vi "Configuration Reference.vi"(8 "Error in":errorcluster, 11 "INL DNL Test in":refnum<class "INL DNL Test.lvclass">) -> (0 "Error out":errorcluster, 2 "VI Ref":refnum<vi>, 3 "INL DNL Test out":refnum<class "INL DNL Test.lvclass">)   [LabVIEW 2020, in "INL DNL Test.lvclass"]
doc: "Runs the configuration page asynchronously."
uses:
  INL DNL Test.lvclass
  Parent/Typedef/LV2 Control.ctl
  Configuration Page.vi
  Parent/Test.lvclass
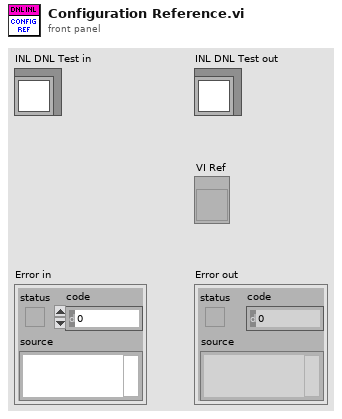
[diagram p1: front panel]
types:
  T1 = typedef "Test.lvclass/LV2 Control.ctl" = enum16{"Home", "Mode", "Config", "Status", "Read"}
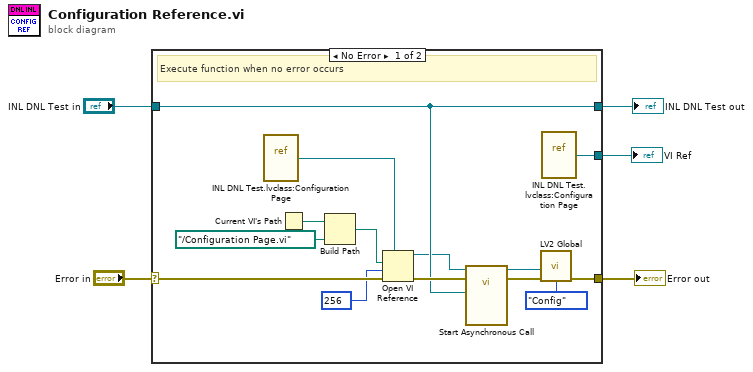
[diagram p0: block diagram]
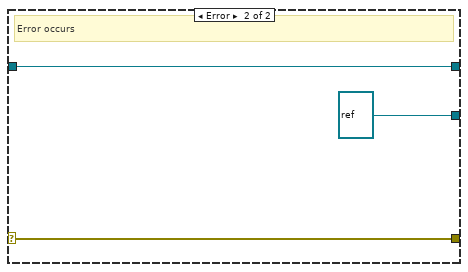
[diagram p2: hidden frame]
diagram:
  n1 = case shown="No Error" "Error in" {
    selector: "Error in" -> [w16 w22]
    tunnel: [w8 w22] -> w4
    tunnel: [w11 w21] -> w2
    tunnel: "INL DNL Test in" -> [w11 w21]
    tunnel: [w19 refnum<vi> refnum] -> w1
    frame No Error {
      # "Execute function when no error occurs"
      n2 = vi-ref "INL DNL Test.lvclass:Configuration Page.vi"() -> (w14:refnum<vi>)
      n3 = Current VI's Path() -> (path=w18:path)
      n4 = Build Path(base path=w18, name or relative path=path "../Configuration Page.vi") -> (appended path=w15:path)
      n5 = Open VI Reference(type specifier VI Refnum (for type only)=w14, vi path=w15, options=256, error in (no error)=w16) -> (vi reference=w10:refnum<vi>, error out=w12:errorcluster)  [unwired: 2 in]
      n6 = call-by-ref "Start Asynchronous Call"(reference=w10, error in=w12, "INL DNL Test.lvclass"=w11) -> (reference out=w6:refnum<vi>, error out=w9:errorcluster)  [unwired: 9 in, 2 out]
      n7 = call "LV2 Global.vi"("Conf In"=w6, "Error In"=w9, "Enum"=LV2_Control."Config") -> ("Error Out"=w8:errorcluster)  [unwired: 8 in, 4 out]
      n8 = vi-ref "INL DNL Test.lvclass:Configuration Page.vi"() -> (w19:refnum<vi>)
    }
    frame Error {
      # "Error occurs"
    }
  }
  "Error out" <- w4
  "INL DNL Test out" <- w2
  "VI Ref" <- w1
